vi "Zamojski_B_1.vi"   [LabVIEW 2020]
uses:
  <vilib>/Platform/TimedLoop/XDataNode/timing_clust.ctl
  <vilib>/Platform/TimedLoop/XDataNode/nitl_modes.ctl
  <vilib>/Platform/TimedLoop/XDataNode/wakeup.ctl
  <vilib>/platform/TimedLoop/XDataNode/XDataNode.xnode
  <vilib>/Platform/TimedLoop/XDataNode/XDNodeRunTimeDep.lvlib
types:
  T1 = typedef "Rendezvous RefNum" = refnum<k1>
  T2 = typedef "Semaphore RefNum" = refnum<k1>
  T3 = typedef "XDNodeRunTimeDep.lvlib/timing_clust.ctl" = cluster{"Expected End [f-1]":u64, "Actual End [f-1]":u64, "Finished Late? [f-1]":bool, "Expected End [i-1]":u64, "Actual End [i-1]":u64, "Finished Late? [i-1]":bool, "Expected Start [i]":u64, "Actual Start [i]":u64, "Expected Start [f]":u64, "Actual Start [f]":u64, "Source Name":string, "Structure Name":string, "Period":i64, "Deadline":i64, "Offset":i64, "Start":i64, "Priority":i32, "Timeout":i32, "Mode":T4, "Wakeup Reason":T5, "Error":errorcluster, "Source Type":string, "Secondary Source Type":string, "Global End Time":u64, "Global Start Time":u64, "Frame Duration":u64, "Iteration Duration":u64, "Assigned CPU":i32, "I/O Scan Engine Mode":u32}
  T4 = typedef "XDNodeRunTimeDep.lvlib/nitl_modes.ctl" = enum32{"No Change", "Process missed periods, maintain original phase", "Discard missed periods, maintain original phase", "Process missed periods, ignore original phase", "Discard missed periods, ignore original phase"}
  T5 = typedef "XDNodeRunTimeDep.lvlib/wakeup.ctl" = enum32{"Normal", "Aborted", "Asynchronous wakeup", "Timing source error", "Timed loop error", "Timeout"}
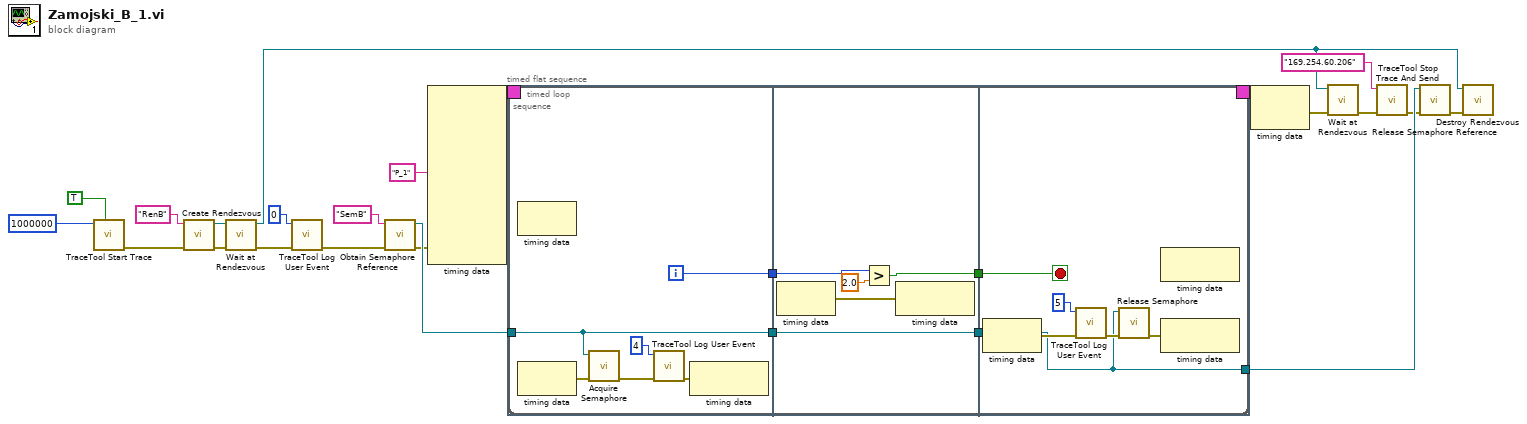
[diagram p0: block diagram]
diagram:
  n1 = call <vilib>:"TraceTool Start Trace.vi"("Detailed Tracing? (F)"=TRUE, "Buffer Size (250000 bytes)"=1000000) -> ("error out"=w2:errorcluster)  [unwired: 8 in, 1 out]
  n2 = call <vilib>:"Create Rendezvous.vi"("error in (no error)"=w2, "name (unnamed)"="RenB") -> ("error out"=w19:errorcluster, "rendezvous"=w21:T1)  [unwired: 3 in, 1 out]
  n3 = call <vilib>:"Wait at Rendezvous.vi"("error in (no error)"=w19, "rendezvous"=w21) -> ("error out"=w18:errorcluster, "rendezvous out"=w5:T1)  [unwired: 3 in, 1 out]
  n4 = call <vilib>:"TraceTool Log User Event.vi"("error in (no error)"=w18, "Event ID (0-255)"=u32 0) -> ("error out"=w17:errorcluster)  [unwired: 9 in]
  n5 = call <vilib>:"Obtain Semaphore Reference.vi"("error in (no error)"=w17, "name (unnamed)"="SemB") -> ("error out"=w1:errorcluster, "semaphore"=w12:T2)  [unwired: 3 in, 1 out]
  n6 = node-c288("P_1" ("Structure Name"), w1) -> (w15:T3)  [unwired: 8 in]
  n7 = timed-loop {
    timing: w15 -> [_]
    timing-out: [_] -> w14
    tunnel: w12 -> [w24]
    tunnel: [w23] -> w11
    i -> [w31]
    stop <- w52 stop-if-true
    n8 = timed-sequence {
      timing: _ -> [_]
      timing-out: _ -> [_]
      tunnel: w24 -> [w28]
      tunnel: [w27] -> w23
      n9 = timed-flat-sequence {
        tunnel: [w32] -> w29
        tunnel: w28 -> [w32]
        tunnel: [w31] -> w26
        tunnel: [w46] -> w30
        tunnel: w29 -> [w46]
        tunnel: w26 -> [w44]
        tunnel: [w43] -> w25
        tunnel: w30 -> [w53]
        tunnel: [w53] -> w27
        tunnel: w25 -> [w52]
        frame #0 {
          n10 = node-c288() -> (w34:errorcluster)  [unwired: 1 in]
          n11 = call <vilib>:"Acquire Semaphore.vi"("error in (no error)"=w34, "semaphore"=w32) -> ("error out"=w35:errorcluster)  [unwired: 3 in, 2 out]
          n12 = call <vilib>:"TraceTool Log User Event.vi"("error in (no error)"=w35, "Event ID (0-255)"=u32 4) -> ("error out"=w33:errorcluster)  [unwired: 9 in]
          n13 = node-c288(w33) -> ()  [unwired: 1 out]
        }
        frame #1 {
          n14 = node-c288() -> (w42:errorcluster)  [unwired: 1 in]
          n15 = Greater?(x=w44, y=2.0) -> (0:w43:bool)
          n16 = node-c288(w42) -> ()  [unwired: 1 out]
        }
        frame #2 {
          n17 = node-c288() -> (w54:errorcluster)  [unwired: 1 in]
          n18 = call <vilib>:"TraceTool Log User Event.vi"("error in (no error)"=w54, "Event ID (0-255)"=u32 5) -> ("error out"=w56:errorcluster)  [unwired: 9 in]
          n19 = call <vilib>:"Release Semaphore.vi"("error in (no error)"=w56, "semaphore"=w53) -> ("error out"=w55:errorcluster)  [unwired: 4 in, 1 out]
          n20 = node-c288(w55) -> ()  [unwired: 1 out]
        }
      }
    }
    n21 = node-c288() -> ()  [unwired: 1 in, 1 out]
    n22 = node-c288() -> ()  [unwired: 1 in, 1 out]
  }
  n23 = node-c288(w14) -> (w4:errorcluster)
  n24 = call <vilib>:"Wait at Rendezvous.vi"("error in (no error)"=w4, "rendezvous"=w5) -> ("error out"=w3:errorcluster)  [unwired: 3 in, 2 out]
  n25 = call <vilib>:"TraceTool Stop Trace And Send.vi"("error in (no error)"=w3, "Trace Host Network Address"="169.254.60.206") -> ("error out"=w7:errorcluster)  [unwired: 9 in]
  n26 = call <vilib>:"Release Semaphore Reference.vi"("error in (no error)"=w7, "semaphore"=w11) -> ("error out"=w10:errorcluster)  [unwired: 8 in, 1 out]
  n27 = call <vilib>:"Destroy Rendezvous.vi"("error in (no error)"=w10, "rendezvous"=w5) -> ()  [unwired: 4 in, 2 out]
